vi "檢測_Match_Sub.vi"(4 "樣本比對參數":T2={"方法"=1, "分數"=800.0, "起始角度"=-5.0, "結束角度"=5.0} {"結束角度" min=-180 max=180 step=5; "方法" items=["快速比對"=1, "精準比對"=2]; "起始角度" min=-180 max=180 step=5}, 6 "ROI Descriptor":T4 {"Contours"."Type" items=["No Selection", "Point", "Line", "Rectangle", "Oval", "Polygon", "Freehand Region", "Annulus", "Unused2", "Unused3", "Broken Line", "Freehand Line", "Rotated Rectangle"]}, 7 "Mode":u16(ring) items=["Find Reference", "Update CoordSys"], 8 "error in (no error)":errorcluster, 9 "Coordinate System In":T3 {"Measurement System"."Axis Reference" items=["Direct", "Indirect"]; "Measurement System"."Angle (deg)" format="%.2f"; "Measurement System"."Origin"."Y" format="%.2f"; "Measurement System"."Origin"."X" format="%.2f"; "Reference System"."Axis Reference" items=["Direct", "Indirect"]; "Reference System"."Angle (deg)" format="%.2f"; "Reference System"."Origin"."Y" format="%.2f"; "Reference System"."Origin"."X" format="%.2f"}, 10 "Template Image":T5, 11 "Image":T5) -> (0 "error out":errorcluster, 1 "Coordinate System Out":T3 {"Measurement System"."Axis Reference" items=["Direct", "Indirect"]; "Measurement System"."Angle (deg)" format="%.2f"; "Measurement System"."Origin"."Y" format="%.2f"; "Measurement System"."Origin"."X" format="%.2f"; "Reference System"."Axis Reference" items=["Direct", "Indirect"]; "Reference System"."Angle (deg)" format="%.2f"; "Reference System"."Origin"."Y" format="%.2f"; "Reference System"."Origin"."X" format="%.2f"}, 2 "Matches (real-world)":T1(array[cluster]) {"Bounding Box"."y" format="%.2f"; "Bounding Box"."x" format="%.2f"; "Score" format="%.2f"; "Scale" format="%.2f"; "Angle" format="%.2f"; "Position"."y" format="%.2f"; "Position"."x" format="%.2f"}, 3 "Image Out":T5)   [LabVIEW 2015]
uses:
  <vilib>/vision/Image Controls.llb/IMAQ Image.ctl
  Setting/0.Control/Setting_Control_Pattern Paremeter.ctl
  <vilib>/vision/NI_Vision_Development_Module.lvlib
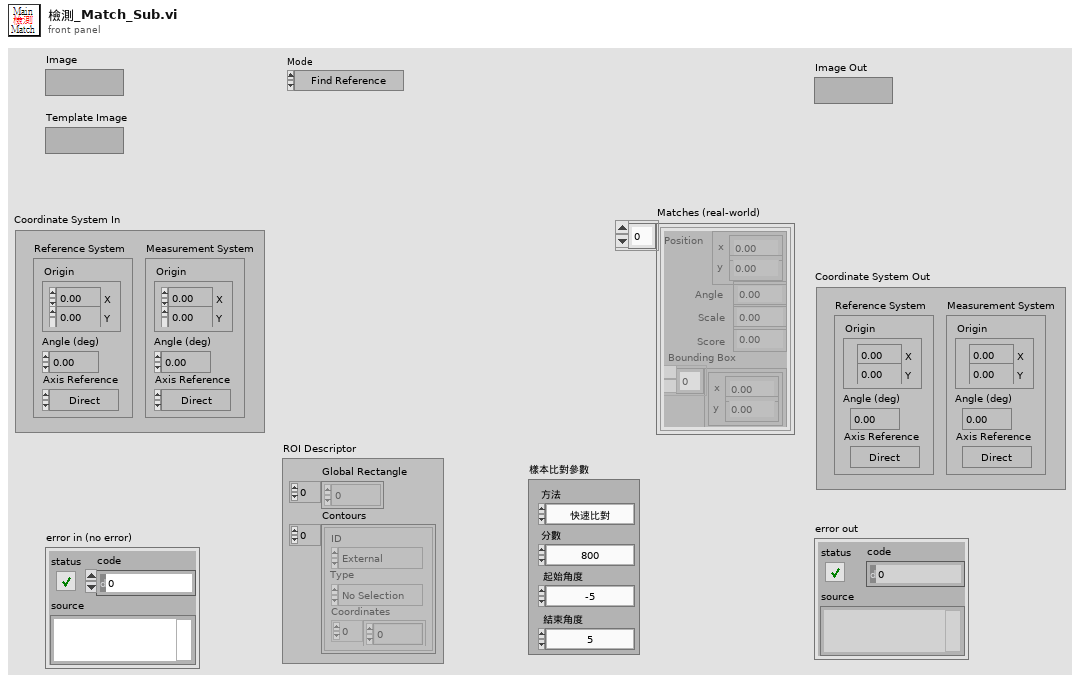
[diagram p1: front panel]
types:
  T1 = cluster{"Position":cluster{"x":sgl, "y":sgl}, "Angle":sgl, "Scale":sgl, "Score":sgl, "Bounding Box":cluster{"x":sgl, "y":sgl}[]}[]
  T2 = typedef "Setting_Control_Pattern Paremeter.ctl" = cluster{"方法":u16, "分數":sgl, "起始角度":sgl, "結束角度":sgl}
  T3 = typedef "IMAQ Coordinate System" = cluster{"Reference System":cluster{"Origin":cluster{"X":sgl, "Y":sgl}, "Angle (deg)":sgl, "Axis Reference":u32}, "Measurement System":cluster{"Origin":cluster{"X":sgl, "Y":sgl}, "Angle (deg)":sgl, "Axis Reference":u32}}
  T4 = typedef "ROI Descriptor" = cluster{"Global Rectangle":i32[], "Contours":cluster{"ID":enum32{"External", "Internal"}, "Type":u32, "Coordinates":i32[]}[]}
  T5 = typedef "IMAQ Image.ctl" = refnum<image>
  T6 = cluster{"Number of Matches Requested":i32, "Minimum Match Score":sgl, "Angle Ranges":cluster{"Start Angle":sgl, "End Angle":sgl}[]}
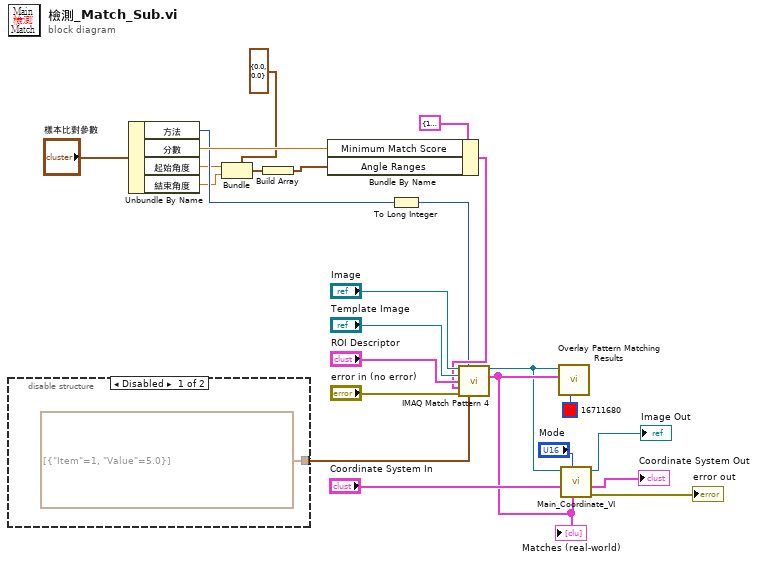
[diagram p0: block diagram]
diagram:
  n1 = disable-structure shown="Disabled" {
    disable-tunnel: [cluster{"Item":u16, "Value":dbl}[] [{"Item"=1, "Value"=5.0}] ("Advanced Options") _] -> w1
    frame Disabled {
    }
    frame Enabled {
    }
  }
  n2 = Unbundle By Name("樣本比對參數") -> ("方法"=w10:u16, "分數"=w12:sgl, "起始角度"=w4:sgl, "結束角度"=w3:sgl)
  n3 = Bundle(cluster=cluster{"Start Angle":sgl, "End Angle":sgl} {"Start Angle"=0.0, "End Angle"=0.0} ("Angle Range"), "Start Angle"=w4, "End Angle"=w3) -> (w11:cluster{"Start Angle":sgl, "End Angle":sgl})
  n4 = Build Array(w11) -> (w5:cluster{"Start Angle":sgl, "End Angle":sgl}[])
  n5 = Bundle By Name(cluster=T6 {"Number of Matches Requested"=1, "Minimum Match Score"=800.0, "Angle Ranges"=[]} ("Parameters"), "Minimum Match Score"=w12, "Angle Ranges"=w5) -> (w9:T6)
  n6 = To Long Integer(number=w10) -> (32bit integer=w7:i32)
  n7 = call "IMAQ Match Pattern 4"("Image"="Image", "Algorithm"=w7, "Template Image"="Template Image", "ROI Descriptor"="ROI Descriptor", "Parameters"=w9, "error in (no error)"="error in (no error)", "Advanced Options"=w1) -> ("Image (duplicate)"=w6:T5, "Matches (real-world)"=w8:T1)  [unwired: 4 in, 3 out]
  "Matches (real-world)" <- w8
  n8 = call "Overlay Pattern Matching Results.vi"("Color"=u32 16711680, "Matches"=w8, "Image"=w6) -> ()  [unwired: 7 in, 2 out]
  n9 = call "Main_Coordinate_VI.vi"("Matches (real-world)"=w8, "Mode"="Mode", "Coordinate System In"="Coordinate System In", "Image In"=w6) -> ("error out"=→"error out":errorcluster, "Coordinate System Out"=→"Coordinate System Out":T3, "Image Out"=→"Image Out":T5)  [unwired: 5 in]
